vi "Teleop.vi"(10 "Match Info":T1={"Autonomous Elapsed Seconds"=0.0, "TeleOp Elapsed Seconds"=0.0, "Disabled Elapsed Seconds"=0.0, "Visited Autonomous"=FALSE, "Visited TeleOp"=FALSE, "Visited Disabled"=FALSE, "Autonomous Settings"={"Autonomous Style"=enum."Independent", "VI Refnum"=refnum}}, 11 "Call Context":T2) -> ()   [LabVIEW 2012]
doc: "This VI is called for each TeleOp packet received from the DS where the robot is not disabled. It is often used to read from the joysticks and update I/O or to update setpoints for timed control loops. It should complete and return within 20 milliseconds or it may miss DS packets."
uses:
  <vilib>/Rock Robotics/WPI/DriverStation/WPI_DriverStationDerivedRobotMode.ctl
  <vilib>/Rock Robotics/WPI/DriverStation/WPI_DriverStationMatch Info.ctl
  Robot Global Data.vi
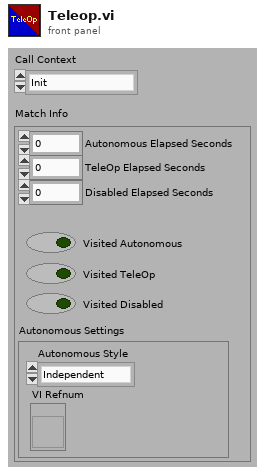
[diagram p1: front panel]
types:
  T1 = typedef "WPI_DriverStationMatch Info.ctl" = cluster{"Autonomous Elapsed Seconds":dbl, "TeleOp Elapsed Seconds":dbl, "Disabled Elapsed Seconds":dbl, "Visited Autonomous":bool, "Visited TeleOp":bool, "Visited Disabled":bool, "Autonomous Settings":cluster{"Autonomous Style":enum16{"Iterative", "Independent"}, "VI Refnum":refnum<vi>}}
  T2 = typedef "WPI_DriverStationDerivedRobotMode.ctl" = enum16{"Init", "Execute", "Stop"}
  T3 = cluster{"Buttons":cluster{"A":bool, "B":bool, "X":bool, "Y":bool, "Left Bumper":bool, "Right Bumper":bool, "Back":bool, "Start":bool, "Left Thumbstick":bool, "Right Thumbstick":bool}, "Axes":cluster{"Left Stick X ":dbl, "Left Stick Y":dbl, "Triggers":dbl, "Right Stick X":dbl, "Right Stick Y":dbl, "D-Pad X":dbl}}
  T4 = cluster{"Joy Stick":cluster{"Secondary":cluster{"Buttons":cluster{"A":bool, "B":bool, "X":bool, "Y":bool, "Left Bumper":bool, "Right Bumper":bool, "Back":bool, "Start":bool, "Left Thumbstick":bool, "Right Thumbstick":bool}, "Axes":cluster{"Left Stick X ":dbl, "Left Stick Y":dbl, "Triggers":dbl, "Right Stick X":dbl, "Right Stick Y":dbl, "D-Pad X":dbl}}, "Primary":cluster{"Buttons":cluster{"A":bool, "B":bool, "X":bool, "Y":bool, "Left Bumper":bool, "Right Bumper":bool, "Back":bool, "Start":bool, "Left Thumbstick":bool, "Right Thumbstick":bool}, "Axes":cluster{"Left Stick X ":dbl, "Left Stick Y":dbl, "Triggers":dbl, "Right Stick X":dbl, "Right Stick Y":dbl, "D-Pad X":dbl}}}, "Arm":cluster{"Arm Set":dbl, "Arm Current":dbl, "At Position?":bool}, "Drive":cluster{"Right":dbl, "Left":dbl}, "Shooter":cluster{"RPM Current":dbl, "RPM Set":dbl, "In Range?":bool}, "Climb State":enum16{"Arm Wait", "Arm Up", "Arm Down", "Arm Attach"}}
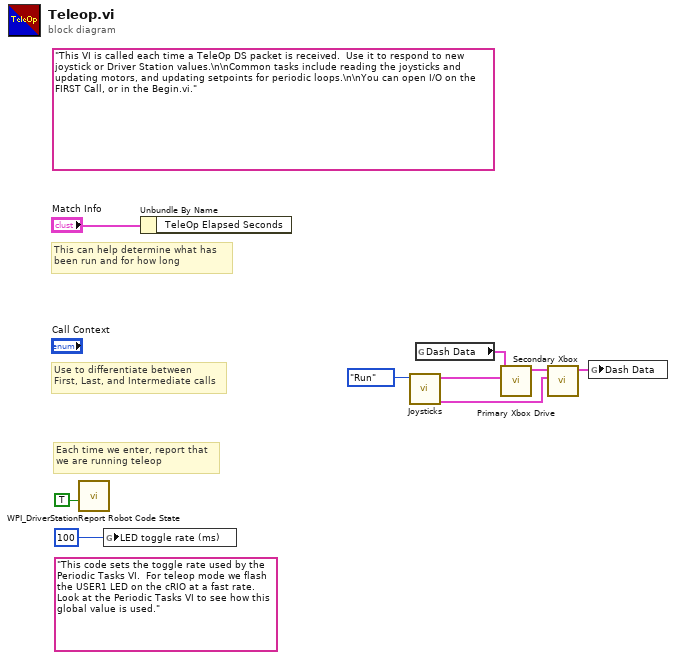
[diagram p0: block diagram]
diagram:
  (unwired) "This code sets the toggle rate used by the Periodic Tasks VI.  For teleop mode we flash the USER1 LED on the cRIO at a fast rate.  Look at the Periodic Tasks VI to see how this global value is used."
  (unwired) "This VI is called each time a TeleOp DS packet is received.  Use it to respond to new joystick or Driver Station values.\n\nCommon tasks include reading the joysticks and updating motors, and updating setpoints for periodic loops.\n\nYou can open I/O on the FIRST Call, or in the Begin.vi."
  # "Each time we enter, report that\nwe are running teleop"
  # "Use to differentiate between\nFirst, Last, and Intermediate calls"
  # "This can help determine what has\nbeen run and for how long"
  n1 = call <vilib>:"WPI_DriverStationReport Robot Code State.vi"("TeleOp"=TRUE ("Autonomous")) -> ()  [unwired: 10 in, 1 out]
  n2 = global write "Robot Global Data.vi" "LED toggle rate (ms)"(u32 100 ("LED ms toggle rate")) -> ()
  n3 = Unbundle By Name("Match Info") -> ()  [unwired: 1 out]
  n4 = call "Joysticks.vi"("Enum"=enum16{"Start", "Run", "End"}."Run") -> ("Secondary"=w5:T3, "Primary"=w2:T3)  [unwired: 9 in]
  n5 = global read "Robot Global Data.vi" "Dash Data"() -> (w4:T4)
  n6 = call "Primary Xbox Drive.vi"("Primary"=w2, "Dash Data in"=w4) -> ("Dash Data out"=w3:T4)  [unwired: 9 in]
  n7 = call "Secondary Xbox.vi"("Secondary"=w5, "Dash Data in"=w3) -> ("Dash Data out"=w1:T4)  [unwired: 9 in]
  n8 = global write "Robot Global Data.vi" "Dash Data"(w1) -> ()
